vi "Configure Device.vi"(8 "error in (no error)":errorcluster, 10 "Max Beams":dbl, 11 "WS1042 in":refnum<class "WS1042.lvclass">) -> (0 "error out":errorcluster, 3 "WS1042 out":refnum<class "WS1042.lvclass">)   [LabVIEW 2020, in "WS1042.lvclass"]
uses:
  WS1042.lvclass
  Toggle 6.lvclass
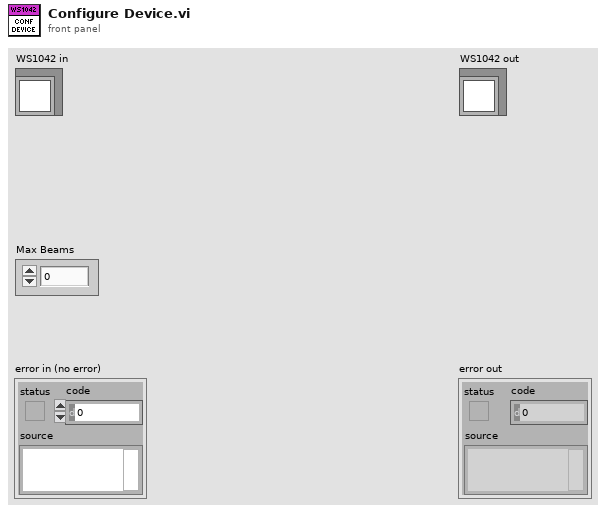
[diagram p1: front panel]
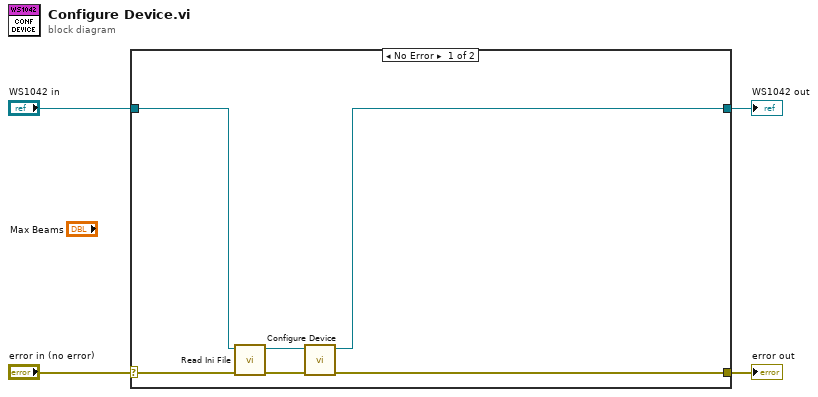
[diagram p0: block diagram]
diagram:
  n1 = case shown="No Error" "error in (no error)" {
    selector: "error in (no error)" -> [w9 w12]
    tunnel: [w5 w12] -> w3
    tunnel: [w6 w11] -> w1
    tunnel: "WS1042 in" -> [w10 w11]
    frame No Error {
      n2 = call "Read Ini File.vi"("error in (no error)"=w9, "WS1042 in"=w10) -> ("error out"=w7:errorcluster, "WS1042 out"=w8:refnum<class "WS1042.lvclass">)  [unwired: 8 in]
      n3 = call-parent "Configure Device.vi"("error in (no error)"=w7, "Toggle 6 in"=w8) -> ("error out"=w5:errorcluster, "Toggle 6 out"=w6:refnum<class "WS1042.lvclass">)  [unwired: 8 in]
    }
    frame Error {
    }
  }
  "error out" <- w3
  "WS1042 out" <- w1
